vi "Get Monitor Bounds of Position.vi"(11 "Position":cluster{"Left":i32, "Top":i32}) -> (3 "Monitor Bounds":T1)   [LabVIEW 2019, in "Peek Window.lvlib"]
uses:
  Peek Window.lvlib
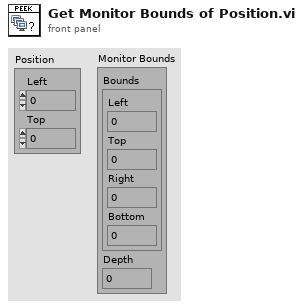
[diagram p1: front panel]
types:
  T1 = cluster{"Bounds":cluster{"Left":i16, "Top":i16, "Right":i16, "Bottom":i16}, "Depth":i16}
  T2 = typedef "LVAllMonitorsDisplayTypeDef.ctl" = cluster{"Bounds":cluster{"Left":i16, "Top":i16, "Right":i16, "Bottom":i16}, "Depth":i16}[]
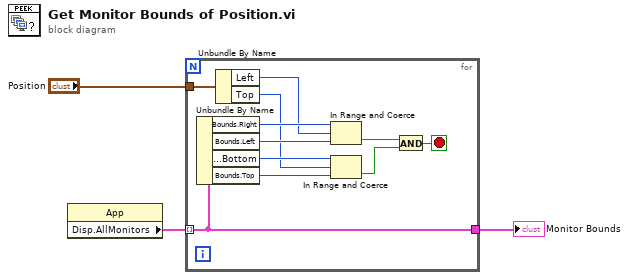
[diagram p0: block diagram]
diagram:
  n1 = property class="App"() -> ("Disp.AllMonitors"=w1:T2)  [unwired: 2 in, 2 out]
  n2 = for {
    tunnel: w1 -> [w9] mode=indexing
    tunnel: "Position" -> [w6]
    tunnel: [w9] -> w3
    stop <- w11 stop-if-true
    n3 = Unbundle By Name(w9) -> ("Bounds.Right"=w7:i16, "Bounds.Left"=w10:i16, "Bounds.Bottom"=w14:i16, "Bounds.Top"=w8:i16)
    n4 = Unbundle By Name(w6) -> ("Left"=w5:i32, "Top"=w4:i32)
    n5 = In Range and Coerce(upper limit=w7, x=w5, lower limit=w10) -> (In Range?=w13:bool)  [unwired: 1 out]
    n6 = In Range and Coerce(upper limit=w14, x=w4, lower limit=w8) -> (In Range?=w12:bool)  [unwired: 1 out]
    n7 = And(x=w13, y=w12) -> (x .and. y?=w11:bool)
  }
  "Monitor Bounds" <- w3
